vi "VG_branche.vi"() -> ()   [LabVIEW 2020]
panel:
  out "Branche":dbl
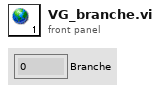
[diagram p1: front panel]
diagram:
